vi "Set Color.vi"(11 "Color in":T1) -> (3 "Color out":T1)   [LabVIEW 2017, in "Simulator Display.xctl"]
uses:
  <vilib>/robotics/Controls/Simulator Display/Simulator Display.xctl
  <vilib>/Utility/miscctls.llb/LVRGBAColorTypeDef.ctl
panel:
  in  "OK Button":bool
  in  "Color":u32(colorbox)
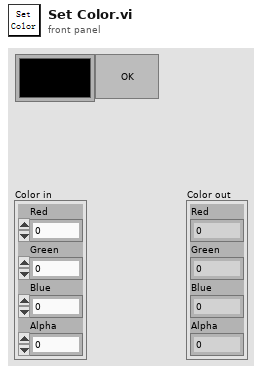
[diagram p1: front panel]
types:
  T1 = typedef "LVRGBAColorTypeDef.ctl" = cluster{"Red":sgl, "Green":sgl, "Blue":sgl, "Alpha":sgl}
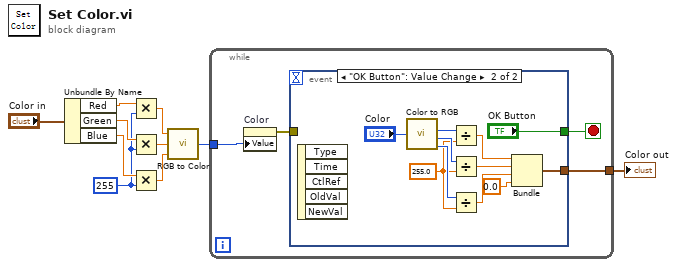
[diagram p0: block diagram]
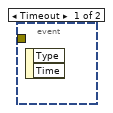
[diagram p2: hidden frame]
diagram:
  w4 = 255 ("y")
  n1 = Unbundle By Name("Color in") -> ("Red"=w8:sgl, "Green"=w6:sgl, "Blue"=w5:sgl)
  n2 = Multiply(x=w8, y=w4) -> (x*y=w7:sgl)
  n3 = Multiply(x=w6, y=w4) -> (x*y=w2:sgl)
  n4 = Multiply(x=w5, y=w4) -> (x*y=w3:sgl)
  n5 = call <vilib>:"RGB to Color.vi"("B"=w3, "G"=w2, "R"=w7) -> ("Color"=w1:u32)
  n6 = while {
    tunnel: [w13] -> w10
    tunnel: w1 -> [w12]
    stop <- w14 stop-if-true
    n7 = property on="Color" class="ColBox"("Value"=w12) -> (error out=w11:errorcluster)  [unwired: 2 in, 1 out]
    n8 = event shown="[1] \"OK Button\": Value Change" {
      selector: _ -> [_ _]
      dyn-events: _ -> [_ _]
      timeout: _ -> [_ _]
      tunnel: [_ "OK Button"] -> w14
      tunnel: [_ w15] -> w13
      tunnel: w11 -> [_ _]
      event Timeout {
        n9 = event-data() -> ()  [unwired: 1 in, 2 out]
      }
      event "OK Button": Value Change {
        w20 = sgl 255.0 ("y")
        n10 = event-data() -> ()  [unwired: 1 in, 5 out]
        n11 = call <vilib>:"Color to RGB.vi"("Color"="Color") -> ("R"=w23:u8, "G"=w22:u8, "B"=w21:u8)  [unwired: 1 out]
        n12 = Divide(x=w23, y=w20) -> (x/y=w17:sgl)
        n13 = Divide(x=w22, y=w20) -> (x/y=w18:sgl)
        n14 = Divide(x=w21, y=w20) -> (x/y=w19:sgl)
        n15 = Bundle(w17, w18, w19, "y"=sgl 0.0) -> (w15:cluster{sgl, sgl, sgl, "y":sgl})  [unwired: 1 in]
      }
    }
  }
  "Color out" <- w10
